vi "Set Node Path.vi"(8 "error in (no error)":errorcluster, 10 "Path in":string, 11 "Node ref in":refnum<k20>) -> (0 "error out":errorcluster, 1 "Found ?":bool, 3 "Node ref out":refnum<k20>)   [LabVIEW 2019, in "LVLIBP CD XML Updater.lvlib" / "Project XML Editor.lvclass"]
uses:
  Project XML Editor.lvclass
  <vilib>/xml/Close Reference(Node).vi
  <vilib>/xml/NI_XML.lvlib
  <resource>/objmgr/DOMUserDefRef.rc
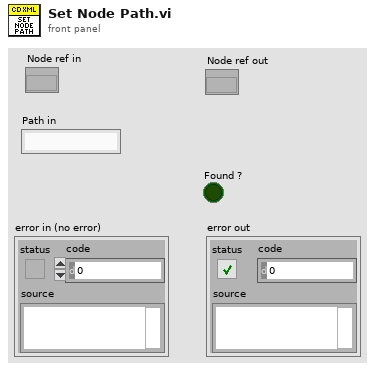
[diagram p1: front panel]
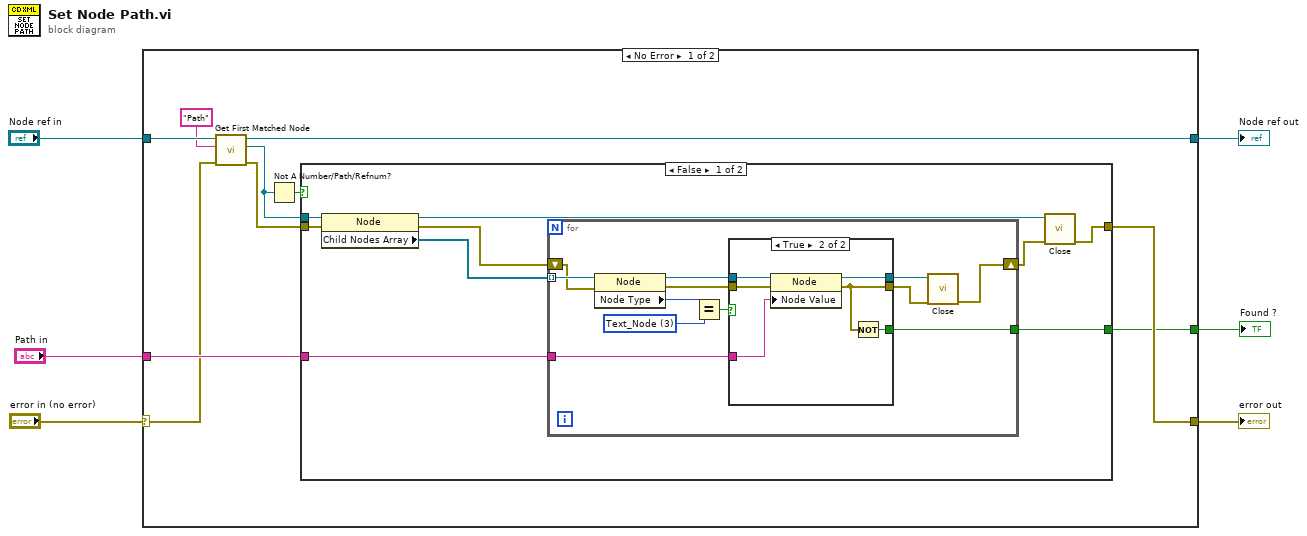
[diagram p0: block diagram]
diagram:
  n1 = case shown="No Error" "error in (no error)" {
    selector: "error in (no error)" -> [w10 w48]
    tunnel: "Node ref in" -> [w16 w47]
    tunnel: [w8 w48] -> w4
    tunnel: [w14 w47] -> w3
    tunnel: "Path in" -> [w11 _]
    tunnel: [w7 _] -> w1
    frame No Error {
      n2 = call <vilib>:"Get First Matched Node.vi"("error in (no error)"=w10, "XPath expression"="Path", "node in"=w16) -> ("error out"=w9:errorcluster, "node result"=w12:refnum<k20>, "node out"=w14:refnum<k20>)  [unwired: 6 in]
      n3 = Not A Number/Path/Refnum?(number/path/refnum=w12) -> (NaN/Path/Refnum?=w13:bool)
      n4 = case shown="False" w13 {
        tunnel: w12 -> [w24 _]
        tunnel: w11 -> [w23 _]
        tunnel: w9 -> [w19 w46]
        tunnel: [w18 w46] -> w8
        tunnel: [w17 _] -> w7
        frame False {
          n5 = property class="Node"(reference=w24, error in=w19) -> (reference out=w22:refnum<k20>, error out=w25:errorcluster, "Child Nodes Array"=w21:refnum<k20>[])
          n6 = for {
            shift-right: [w28] -> w20
            shift-left: w25 -> [w36]
            tunnel: w21 -> [w37] mode=indexing
            tunnel: w23 -> [w27]
            tunnel: [w26] -> w17
            w34 = 3 items=["Element_Node"=1, "Attribute_Node"=2, "Text_Node"=3, "CDATASection_Node"=4, "EntityReference_Node"=5, "Entity_Node"=6, "ProcessingInstruction_Node"=7, "Comment_Node"=8, "Document_Node"=9, "DocumentType_Node"=10, "DocumentFragment_Node"=11, "Notation_Node"=12] ("Node Type")
            n7 = property class="Node"(reference=w37, error in=w36) -> (reference out=w32:refnum<k20>, error out=w31:errorcluster, "Node Type"=w35:i32)
            n8 = Equal?(x=w35, y=w34) -> (x = y?=w33:bool)
            n9 = case shown="True" w33 {
              tunnel: w32 -> [w39 w45]
              tunnel: w31 -> [w38 w44]
              tunnel: [w39 w43] -> w30
              tunnel: [w38 w41] -> w29
              tunnel: w27 -> [_ w42]
              tunnel: [_ w40] -> w26
              frame False {
              }
              frame True {
                n10 = property class="Node"(reference=w45, error in=w44, "Node Value"=w42) -> (reference out=w43:refnum<k20>, error out=w41:errorcluster)
                n11 = Not(x=w41) -> (.not. x?=w40:bool)
              }
            }
            n12 = call-poly <vilib>:"Close.vi"("error in (no error)"=w29, "node"=w30) -> ("error out"=w28:errorcluster)  [unwired: 7 out]
          }
          n13 = call-poly <vilib>:"Close.vi"("error in (no error)"=w20, "node"=w22) -> ("error out"=w18:errorcluster)  [unwired: 7 out]
        }
        frame True {
        }
      }
    }
    frame Error {
    }
  }
  "error out" <- w4
  "Node ref out" <- w3
  "Found ?" <- w1
